vi "Led Matrix Control.vi"(0 "LED Location":u8, 1 "MCU addresses":T1="D", 2 "Red":u8(slide)=255 scale=0.0..255.0, 3 "Green":u8(slide)=255 scale=0.0..255.0, 4 "Blue":u8(slide)=255 scale=0.0..255.0, 8 "Send To MCU":bool, 9 "Close Tab":bool) -> (5 "STOP ALL OUT":bool)   [LabVIEW 2016]
doc: "This SubVI is for controlling the RGB led from LabVIEW in the various rooms.\nChoose perfered colour configuration and press send.\nPlace it in a Case and it will pop up when that case is selected."
uses:
  Typedef/MCU_addresses.ctl
  Typedef/Type_of_message_to_MCU.ctl
  Typedef/Type_of_request.ctl
panel:
  in  "STOP ALL":bool
  out "error out":errorcluster
  out "Converted Message":string
  out "Byte array has been sent":u8[](array[numeric])
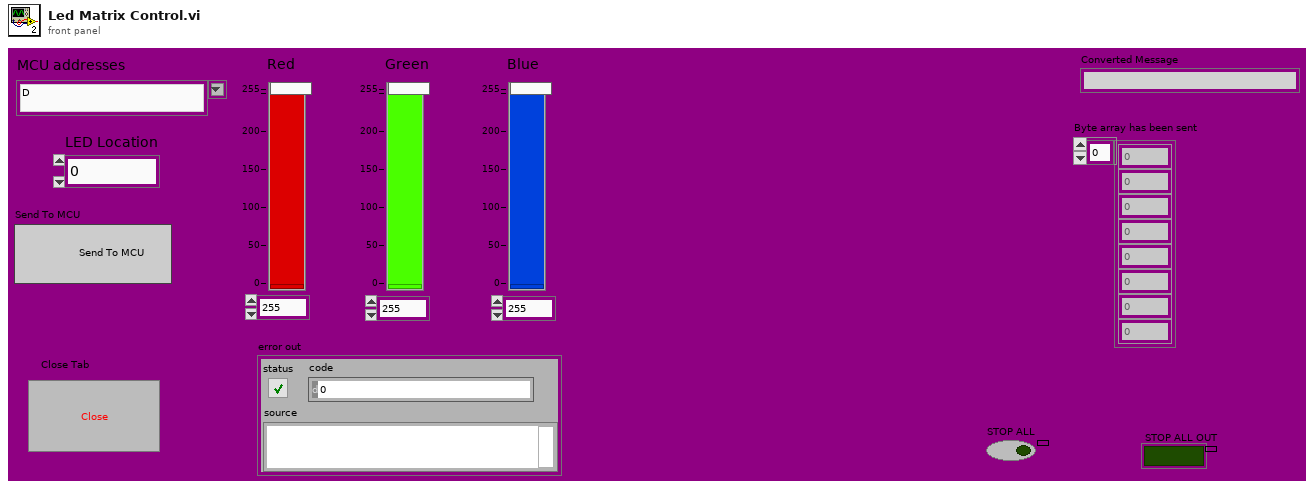
[diagram p1: front panel]
types:
  T1 = typedef "MCU_addresses.ctl" = string
  T2 = typedef "Type_of_message_to_MCU.ctl" = enum16{"Non", "Alarm", "Error", "Time and Date", "Status", "Request", "Command"}
  T3 = typedef "Type_of_request.ctl" = u8
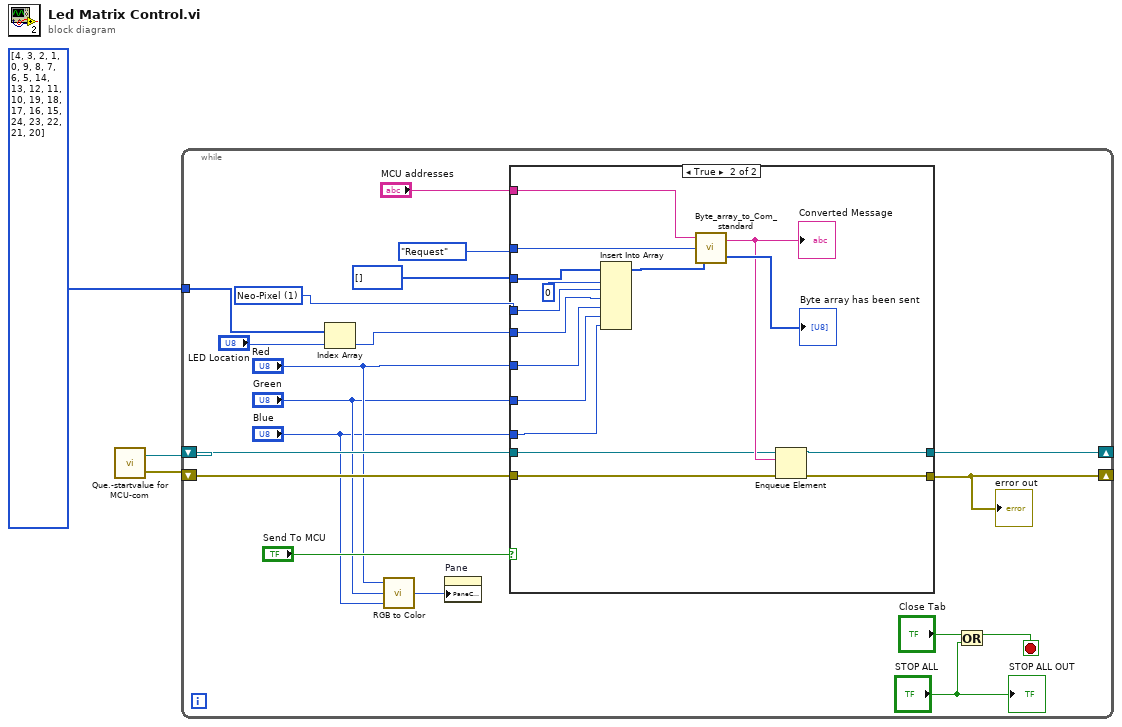
[diagram p0: block diagram]
diagram:
  n1 = call "Que.-startvalue for MCU-com.vi"() -> ("error out"=w2:errorcluster, "queue out"=w3:refnum<queue>)  [unwired: 2 in]
  n2 = while {
    shift-right: [w14] -> _
    shift-left: w3 -> [w17]
    shift-right: [w15] -> _
    shift-left: w2 -> [w16]
    tunnel: i32[] [4, 3, 2, 1, 0, 9, 8, 7, 6, 5, 14, 13, 12, 11, 10, 19, 18, 17, 16, 15, 24, 23, 22, 21, 20] -> [w5]
    stop <- w9 stop-if-true
    w7 = T3 1 items=["Unknown", "Neo-Pixel", "Fan Control", "Heat Control", "Display Text"] ("Ring")
    n3 = Index Array(array=w5, index="LED Location") -> (element=w4:i32)
    n4 = call <vilib>:"RGB to Color.vi"("B"="Blue", "G"="Green", "R"="Red") -> ("Color"=w13:u32)
    n5 = property on="Pane" class="Pane"("PaneColor"=w13) -> ()  [unwired: 2 in, 2 out]
    n6 = case shown="True" "Send To MCU" {
      tunnel: w4 -> [_ w39]
      tunnel: "Red" -> [_ w38]
      tunnel: "Green" -> [_ w37]
      tunnel: "Blue" -> [_ w36]
      tunnel: "MCU addresses" -> [_ w35]
      tunnel: Type_of_message_to_MCU."Request" ("Types of Data") -> [_ w34]
      tunnel: u8[] [] -> [_ w33]
      tunnel: w17 -> [w23 w29]
      tunnel: w16 -> [w24 w28]
      tunnel: [w24 w26] -> w15
      tunnel: [w23 w27] -> w14
      tunnel: w7 -> [_ w25]
      frame False {
      }
      frame True {
        n7 = Insert Into Array(array=w33, index=0, new element #1=w25, new element #2=w39, new element #3=w38, new element #4=w37, new element #5=w36) -> (w32:u8[])
        n8 = call "Byte_array_to_Com_standard.vi"("Payload  Byte to be sent"=w32, "Types of Data"=w34, "MCU Address to be sent"=w35) -> ("Byte array has been sent"=→"Byte array has been sent":u8[], "Converted Message"=w30:string)
        "Converted Message" <- w30
        n9 = Enqueue Element(queue=w29, element=w30, error in (no error)=w28) -> (queue out=w27:refnum<queue>, error out=w26:errorcluster)  [unwired: 1 in, 1 out]
      }
    }
    "error out" <- w15
    n10 = Or(x="Close Tab", y="STOP ALL") -> (x .or. y?=w9:bool)
    "STOP ALL OUT" <- "STOP ALL"
  }
